vi "Migrate Measurement Dependencies.vi"(0 "Project path":path, 1 "Init":T1[](array[typedef]), 5 "Measurement path":path, 7 "Dependencies path":path[](array[path]), 9 "Plug-in name":string, 11 "error in (no error)":errorcluster) -> (4 "Project reference":refnum<vi>, 6 "MeasurementCore reference":refnum<vi>, 8 "Outside items":string[](array[string]), 15 "error out":errorcluster)   [LabVIEW 2021, in "Multiple Migrator.lvlib"]
uses:
  Multiple Migrator.lvlib
  controls/Library Info.ctl
  Generator/_InstrumentStudio Plug-In Editor/InstrumentStudio Plug-In Editor.lvlib
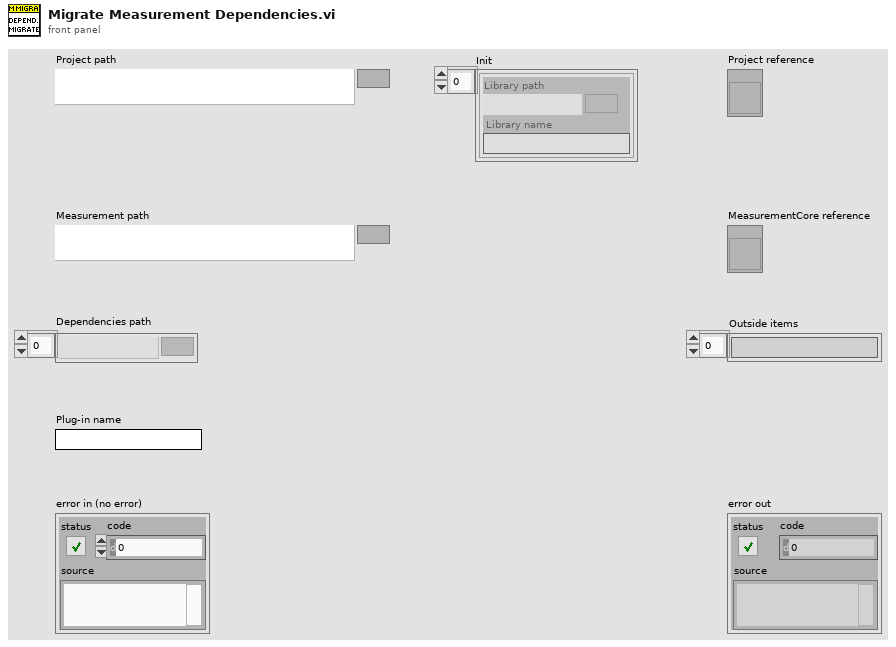
[diagram p1: front panel]
types:
  T1 = typedef "Multiple Migrator.lvlib/Library Info.ctl" = cluster{"Library path":path, "Library name":string}
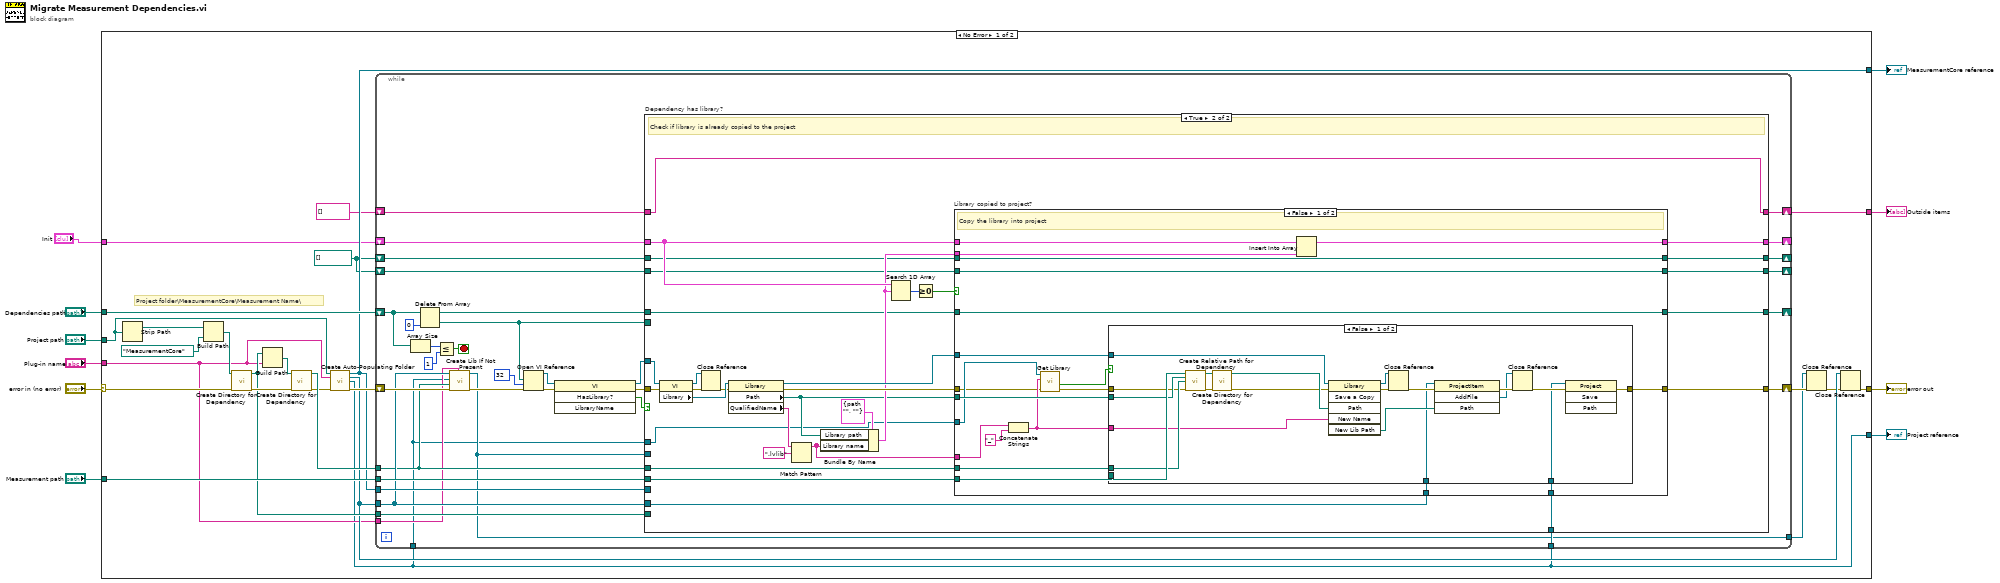
[diagram p0: block diagram]
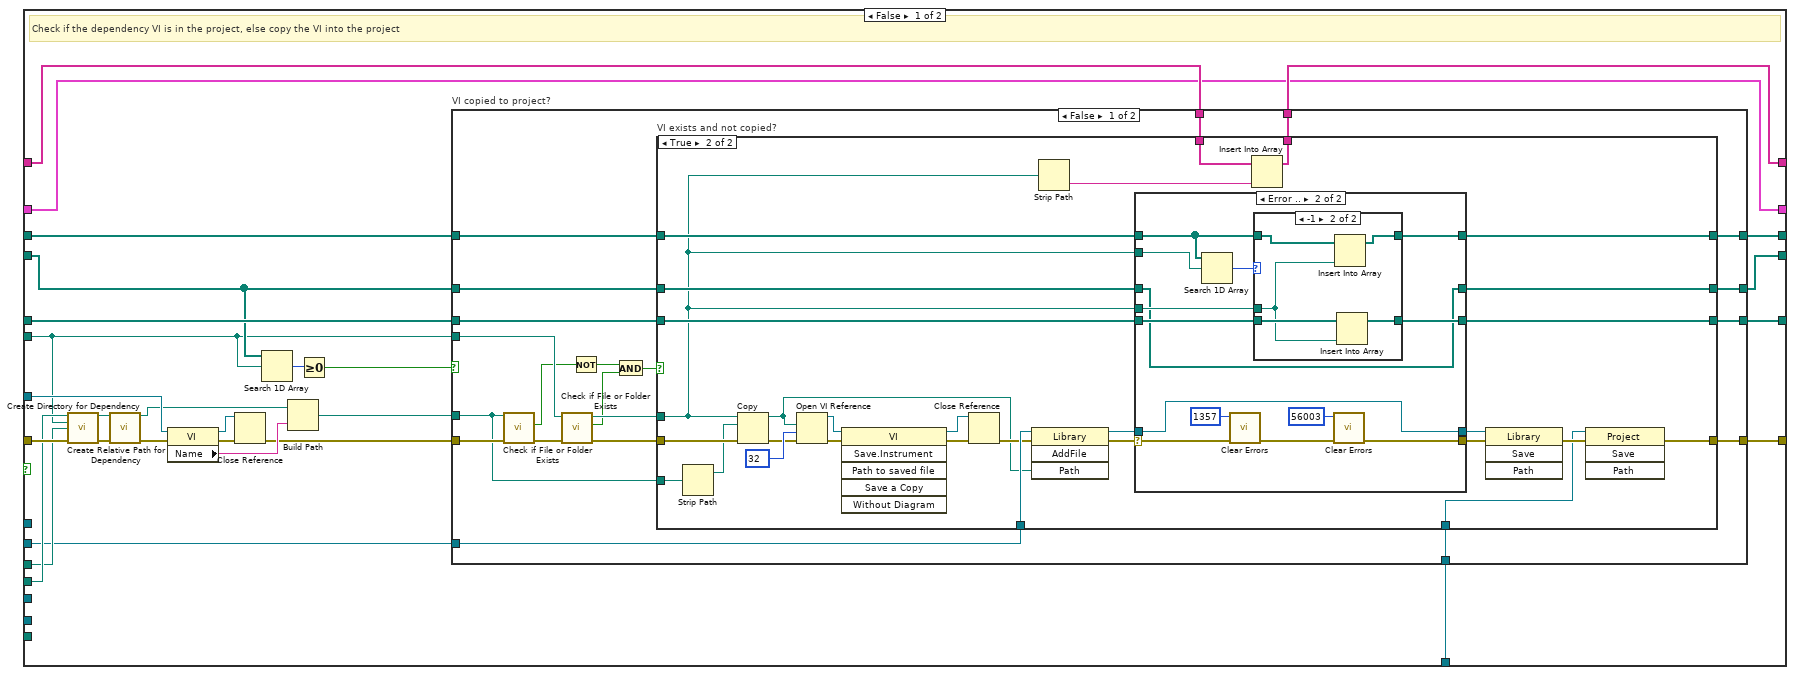
[diagram p2: hidden frame]
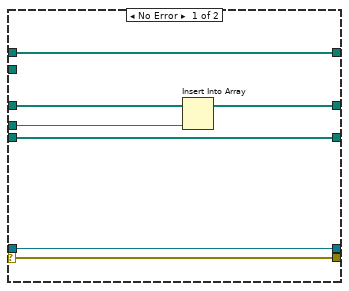
[diagram p4: hidden frame]
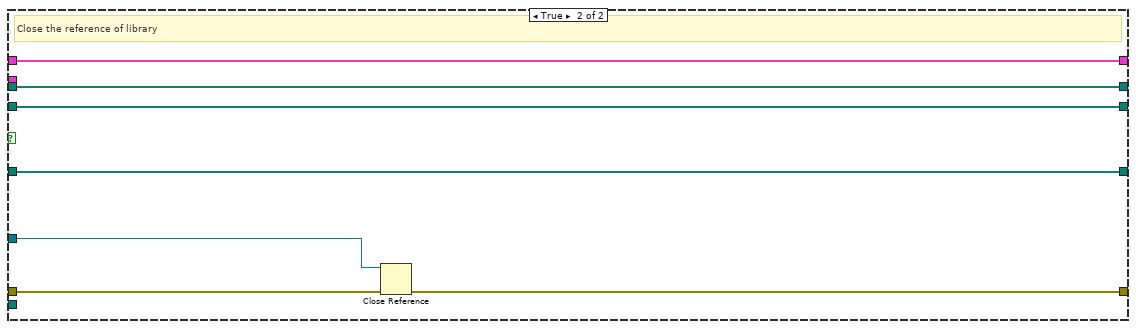
[diagram p8: hidden frame]
diagram:
  n1 = case shown="No Error" "error in (no error)" {
    selector: "error in (no error)" -> [w27 w265]
    tunnel: [w20 w265] -> w9
    tunnel: "Project path" -> [w26 _]
    tunnel: "Measurement path" -> [w31 _]
    tunnel: "Dependencies path" -> [w35 _]
    tunnel: "Plug-in name" -> [w18 _]
    tunnel: [w22 _] -> w4
    tunnel: [w15 _] -> w3
    tunnel: [w16 _] -> w2
    tunnel: "Init" -> [w11 _]
    frame No Error {
      w12 = path[] []
      # "Project folder\\MeasurementCore\\Measurement Name\\"
      n2 = Strip Path(path=w26) -> (stripped path=w30:path)  [unwired: 1 out]
      n3 = Build Path(base path=w30, name or relative path=path "MeasurementCore") -> (appended path=w28:path)
      n4 = call "Create Directory for Dependency.vi"("Directory path"=w28, "error in (no error)"=w27) -> ("Directory path out"=w21:path, "error out"=w25:errorcluster)  [unwired: 12 in]
      n5 = Build Path(base path=w21, name or relative path=w18) -> (appended path=w34:path)
      n6 = call "Create Directory for Dependency.vi"("Directory path"=w34, "error in (no error)"=w25) -> ("Directory path out"=w33:path, "error out"=w24:errorcluster)  [unwired: 12 in]
      n7 = call "Create Auto-Populating Folder.vi"("Project path"=w26, "Plug-in name"=w18, "error in (no error)"=w24) -> ("MeasurementCore reference"=w22:refnum<vi>, "Folder reference"=w19:refnum<vi>, "Project reference"=w15:refnum<vi>, "error out"=w23:errorcluster)  [unwired: 9 in]
      n8 = while {
        shift-right: [w57] -> w32
        shift-left: w23 -> [w45]
        shift-right: [w50] -> _
        shift-left: w35 -> [w67]
        tunnel: w33 -> [w42]
        shift-right: [w56] -> _
        shift-left: w11 -> [w59]
        tunnel: w31 -> [w55]
        shift-right: [w52] -> _
        shift-left: w12 -> [w53]
        tunnel: w22 -> [w49]
        tunnel: w21 -> [w48]
        tunnel: w19 -> [w43]
        tunnel: w18 -> [w41]
        shift-right: [w46] -> w16
        shift-left: string[] [] -> [w47]
        tunnel: w15 -> [w36]
        tunnel: w15 -> [w40]
        shift-right: [w39] -> _
        shift-left: w12 -> [w38]
        tunnel: [w37] -> w13
        stop <- w66 stop-if-true
        n9 = Array Size(array=w67) -> (size(s)=w69:i32)
        n10 = Delete From Array(array=w67, index=0) -> (deleted portion=w54:path, array with subset deleted=w51:path[])  [unwired: 1 in]
        n11 = Less Or Equal?(x=w69, y=1) -> (x <= y?=w66:bool)
        n12 = call "Create Lib If Not Present.vi"("Plug-in name"=w41, "error in (no error)"=w45, "DestDirectory"=w42, "ProjectRef"=w36, "VirtualFolderRef"=w43) -> ("error out"=w44:errorcluster, "Library Refnum"=w37:refnum<vi>)  [unwired: 5 in]
        n13 = Open VI Reference(vi path=w54, options=32, error in (no error)=w44) -> (vi reference=w63:refnum<vi>, error out=w65:errorcluster)  [unwired: 3 in]
        n14 = invoke class="VI" method="HasLibrary?"(reference=w63, error in=w65) -> (reference out=w60:refnum<vi>, error out=w61:errorcluster, "Has Library?"=w62:bool)  [unwired: 2 in, 1 out]
        n15 = case "Dependency has library?" shown="True" w62 {
          tunnel: w61 -> [w96 w215]
          tunnel: w60 -> [w92 w216]
          tunnel: w59 -> [w73 w203]
          tunnel: [w87 w204] -> w57
          tunnel: [w73 w202] -> w56
          tunnel: w55 -> [w95 w200]
          tunnel: w42 -> [w78 w198]
          tunnel: w54 -> [w82 _]
          tunnel: w53 -> [w83 w195]
          tunnel: [w77 w194] -> w52
          tunnel: w51 -> [w86 w193]
          tunnel: [w85 w192] -> w50
          tunnel: w49 -> [_ _]
          tunnel: w48 -> [_ _]
          tunnel: w43 -> [_ w191]
          tunnel: w47 -> [w75 w190]
          tunnel: [w74 w190] -> w46
          tunnel: w37 -> [w76 _]
          tunnel: w40 -> [w70 w189]
          tunnel: [w72 w187] -> w39
          tunnel: w38 -> [w71 w188]
          tunnel: w36 -> [_ w186]
          frame False {
            # "Check if the dependency VI is in the project, else copy the VI into the project"
            n16 = call "Create Relative Path for Dependency.vi"("Old Main Path"=w95, "Old Dependency Path"=w82, "New Dir"=w78, "error in (no error)"=w96) -> ("Directory"=w94:path, "error out"=w97:errorcluster)  [unwired: 10 in]
            n17 = call "Create Directory for Dependency.vi"("Directory path"=w94, "error in (no error)"=w97) -> ("Directory path out"=w84:path, "error out"=w93:errorcluster)  [unwired: 12 in]
            n18 = property class="VI"(reference=w92, error in=w93) -> (reference out=w88:refnum<vi>, error out=w91:errorcluster, "Name"=w90:string)
            n19 = Close Reference(reference=w88, error in (no error)=w91) -> (error out=w89:errorcluster)
            n20 = Search 1D Array(1D array=w83, element=w82) -> (index of element=w81:i32)  [unwired: 1 in]
            n21 = Build Path(base path=w84, name or relative path=w90) -> (appended path=w80:path)
            n22 = Greater Or Equal To 0?(x=w81) -> (x >= 0?=w79:bool)
            n23 = case "VI copied to project?" shown="False" w79 {
              tunnel: w89 -> [w118 w185]
              tunnel: w82 -> [w117 _]
              tunnel: [w114 w185] -> w87
              tunnel: w83 -> [w113 w184]
              tunnel: [w112 w184] -> w77
              tunnel: w80 -> [w108 _]
              tunnel: w86 -> [w111 w183]
              tunnel: [w110 w183] -> w85
              tunnel: w75 -> [w103 w182]
              tunnel: [w102 w182] -> w74
              tunnel: w76 -> [w101 _]
              tunnel: [w100 w181] -> w72
              tunnel: w71 -> [w99 w181]
              tunnel: w70 -> [w98 _]
              frame False {
                n24 = call <vilib>:"Check if File or Folder Exists.vi"("error in (no error)"=w118, "path"=w108) -> ("error out"=w109:errorcluster, "file or folder exists?"=w107:bool)  [unwired: 7 in, 1 out]
                n25 = call <vilib>:"Check if File or Folder Exists.vi"("error in (no error)"=w109, "path"=w117) -> ("error out"=w116:errorcluster, "file or folder exists?"=w105:bool, "dup path"=w115:path)  [unwired: 7 in]
                n26 = Not(x=w107) -> (.not. x?=w106:bool)
                n27 = And(x=w106, y=w105) -> (x .and. y?=w104:bool)
                n28 = case "VI exists and not copied?" shown="True" w104 {
                  tunnel: w116 -> [w123 w152]
                  tunnel: w115 -> [_ w132]
                  tunnel: [w123 w134] -> w114
                  tunnel: w113 -> [w122 w151]
                  tunnel: [w122 w150] -> w112
                  tunnel: w108 -> [_ w147]
                  tunnel: w111 -> [w121 w136]
                  tunnel: [w121 w135] -> w110
                  tunnel: w103 -> [w120 w146]
                  tunnel: [w120 w144] -> w102
                  tunnel: w101 -> [_ w143]
                  tunnel: [w119 w142] -> w100
                  tunnel: w99 -> [w119 w141]
                  tunnel: w98 -> [_ w133]
                  frame False {
                  }
                  frame True {
                    n29 = Strip Path(path=w147) -> (stripped path=w149:path)  [unwired: 1 out]
                    n30 = Copy(8:w152, 10:w149, 11:w132) -> (0:w126:errorcluster, 3:w124:path)  [unwired: 2 in, 1 out]
                    n31 = Open VI Reference(vi path=w124, options=32, error in (no error)=w126) -> (vi reference=w129:refnum<vi>, error out=w130:errorcluster)  [unwired: 3 in]
                    n32 = invoke class="VI" method="Save.Instrument"(reference=w129, error in=w130) -> (reference out=w127:refnum<vi>, error out=w128:errorcluster)  [unwired: 4 in, 4 out]
                    n33 = Close Reference(reference=w127, error in (no error)=w128) -> (error out=w125:errorcluster)
                    n34 = invoke class="Library" method="AddFile"(reference=w143, error in=w125, "Path"=w124) -> (reference out=w140:refnum<vi>, error out=w139:errorcluster)  [unwired: 1 in, 2 out]
                    n35 = Strip Path(path=w132) -> (name=w145:string)  [unwired: 1 out]
                    n36 = case shown="Error .." w139 {
                      selector: w139 -> [w154 w173]
                      tunnel: w151 -> [w159 w160]
                      tunnel: [w158 w160] -> w150
                      tunnel: w132 -> [w157 w163]
                      tunnel: [w156 w164] -> w142
                      tunnel: w141 -> [w156 w165]
                      tunnel: [w155 w162] -> w137
                      tunnel: w140 -> [w155 w162]
                      tunnel: [w154 w171] -> w138
                      tunnel: w136 -> [w153 w167]
                      tunnel: [w153 w166] -> w135
                      tunnel: w132 -> [_ w168]
                      frame No Error {
                        n37 = Insert Into Array(array=w159, new element=w157) -> (w158:path[])  [unwired: 1 in]
                      }
                      frame Error {
                        n38 = Search 1D Array(1D array=w165, element=w168) -> (index of element=w161:i32)  [unwired: 1 in]
                        n39 = call <vilib>:"Clear Errors.vi"("error in (no error)"=w173, "specific error code to clear (0: all)"=1357) -> ("error out"=w172:errorcluster)  [unwired: 4 in, 1 out]
                        n40 = case shown="-1" w161 {
                          tunnel: w167 -> [w174 w180]
                          tunnel: [w174 w179] -> w166
                          tunnel: w165 -> [w175 w178]
                          tunnel: [w175 w177] -> w164
                          tunnel: w163 -> [_ w176]
                          frame Default {
                          }
                          frame -1 {
                            n41 = Insert Into Array(array=w178, new element=w176) -> (w177:path[])  [unwired: 1 in]
                            n42 = Insert Into Array(array=w180, new element=w176) -> (w179:path[])  [unwired: 1 in]
                          }
                        }
                        n43 = call <vilib>:"Clear Errors.vi"("error in (no error)"=w172, "specific error code to clear (0: all)"=56003) -> ("error out"=w171:errorcluster)  [unwired: 4 in, 1 out]
                      }
                    }
                    n44 = Insert Into Array(array=w146, new element=w145) -> (w144:string[])  [unwired: 1 in]
                    n45 = invoke class="Library" method="Save"(reference=w137, error in=w138) -> (error out=w148:errorcluster)  [unwired: 2 in, 3 out]
                    n46 = invoke class="Project" method="Save"(reference=w133, error in=w148) -> (error out=w134:errorcluster)  [unwired: 2 in, 3 out]
                  }
                }
              }
              frame True {
              }
            }
          }
          frame True {
            # "Check if library is already copied to the project"
            n47 = property class="VI"(reference=w216, error in=w215) -> (reference out=w206:refnum<vi>, error out=w214:errorcluster, "Library"=w213:refnum<vi>)
            n48 = Close Reference(reference=w206, error in (no error)=w214) -> (error out=w207:errorcluster)
            n49 = property class="Library"(reference=w213, error in=w207) -> (reference out=w205:refnum<vi>, error out=w208:errorcluster, "Path"=w199:path, "QualifiedName"=w209:string)
            n50 = Match Pattern(string=w209, regular expression=".lvlib") -> (before substring=w196:string)  [unwired: 1 in, 3 out]
            n51 = Bundle By Name(cluster=T1 {"Library path"=path "", "Library name"=""} ("Cluster"), "Library path"=w199, "Library name"=w196) -> (w201:T1)
            n52 = Search 1D Array(1D array=w203, element=w201) -> (index of element=w211:i32)  [unwired: 1 in]
            n53 = Greater Or Equal To 0?(x=w211) -> (x >= 0?=w210:bool)
            n54 = case "Library copied to project?" shown="False" w210 {
              tunnel: w208 -> [w218 w263]
              tunnel: w205 -> [w230 w264]
              tunnel: [w224 w262] -> w204
              tunnel: w203 -> [w236 w261]
              tunnel: [w235 w261] -> w202
              tunnel: w201 -> [w234 _]
              tunnel: w200 -> [w233 _]
              tunnel: w199 -> [w232 _]
              tunnel: w198 -> [w231 _]
              tunnel: w196 -> [w226 _]
              tunnel: w195 -> [w229 w260]
              tunnel: [w229 w260] -> w194
              tunnel: [w228 w259] -> w192
              tunnel: w193 -> [w228 w259]
              tunnel: w191 -> [w227 _]
              tunnel: w189 -> [w223 _]
              tunnel: [w222 w258] -> w187
              tunnel: w188 -> [w222 w258]
              tunnel: w186 -> [w221 _]
              frame False {
                # "Copy the library into project"
                n55 = Concatenate Strings(w226, "_" ("string")) -> (w220:string)
                n56 = call "Get Library.vi"("error in"=w218, "library name"=w220, "project ref"=w221) -> ("error out"=w219:errorcluster, "found"=w217:bool)  [unwired: 5 in, 2 out]
                n57 = case shown="False" w217 {
                  tunnel: w233 -> [w254 _]
                  tunnel: w232 -> [w253 _]
                  tunnel: w231 -> [w252 _]
                  tunnel: w230 -> [w248 _]
                  tunnel: w227 -> [w241 _]
                  tunnel: [w240 w257] -> w224
                  tunnel: w223 -> [w239 _]
                  tunnel: w220 -> [w238 _]
                  tunnel: w219 -> [w237 w257]
                  frame False {
                    n58 = call "Create Relative Path for Dependency.vi"("Old Main Path"=w254, "Old Dependency Path"=w253, "New Dir"=w252, "error in (no error)"=w237) -> ("Directory"=w250:path, "error out"=w251:errorcluster)  [unwired: 10 in]
                    n59 = call "Create Directory for Dependency.vi"("Directory path"=w250, "error in (no error)"=w251) -> ("Directory path out"=w249:path, "error out"=w247:errorcluster)  [unwired: 12 in]
                    n60 = invoke class="Library" method="Save a Copy"(reference=w248, error in=w247, "Path"=w249, "New Name"=w238) -> (reference out=w255:refnum<vi>, error out=w256:errorcluster, "New Lib Path"=w244:path)  [unwired: 2 in, 3 out]
                    n61 = Close Reference(reference=w255, error in (no error)=w256) -> (error out=w246:errorcluster)
                    n62 = invoke class="ProjectItem" method="AddFile"(reference=w241, error in=w246, "Path"=w244) -> (error out=w245:errorcluster, "AddFile"=w242:refnum<vi>)  [unwired: 1 in, 2 out]
                    n63 = Close Reference(reference=w242, error in (no error)=w245) -> (error out=w243:errorcluster)
                    n64 = invoke class="Project" method="Save"(reference=w239, error in=w243) -> (error out=w240:errorcluster)  [unwired: 2 in, 3 out]
                  }
                  frame True {
                  }
                }
                n65 = Insert Into Array(array=w236, new element=w234) -> (w235:T1[])  [unwired: 1 in]
              }
              frame True {
                # "Close the reference of library"
                n66 = Close Reference(reference=w264, error in (no error)=w263) -> (error out=w262:errorcluster)
              }
            }
          }
        }
      }
      n67 = Close Reference(reference=w13, error in (no error)=w32) -> (error out=w14:errorcluster)
      n68 = Close Reference(reference=w19, error in (no error)=w14) -> (error out=w20:errorcluster)
    }
    frame Error {
    }
  }
  "error out" <- w9
  "MeasurementCore reference" <- w4
  "Project reference" <- w3
  "Outside items" <- w2
